vi "intersecAreaCirc.vi"(5 "theta":dbl, 6 "Recuo":dbl=130.0, 8 "error in (no error)":errorcluster, 9 "Ball/Enemy\nPosition":dbl[](array[numeric]), 10 "Game":refnum<class "Game.lvclass">, 11 "Utilities in":refnum<class "Utilities.lvclass">) -> (0 "error out":errorcluster, 2 "Position":dbl[](array[numeric]), 3 "Utilities out":refnum<class "Utilities.lvclass">)   [LabVIEW 2023, in "Utilities.lvclass"]
uses:
  Utilities.lvclass
  Game_class/Game.lvclass
  Game_class/Game.lvclass/Game.ctl
  Game_class/Read FieldRef.vi
  Field_class/Field.lvclass
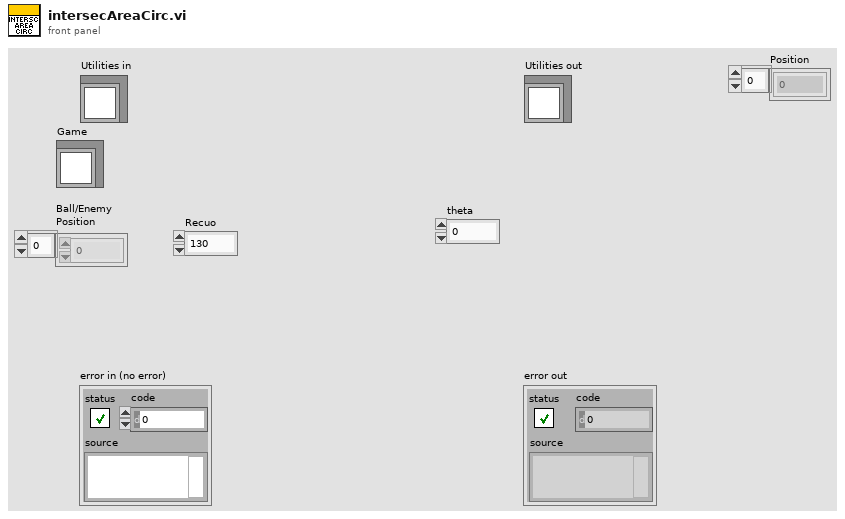
[diagram p1: front panel]
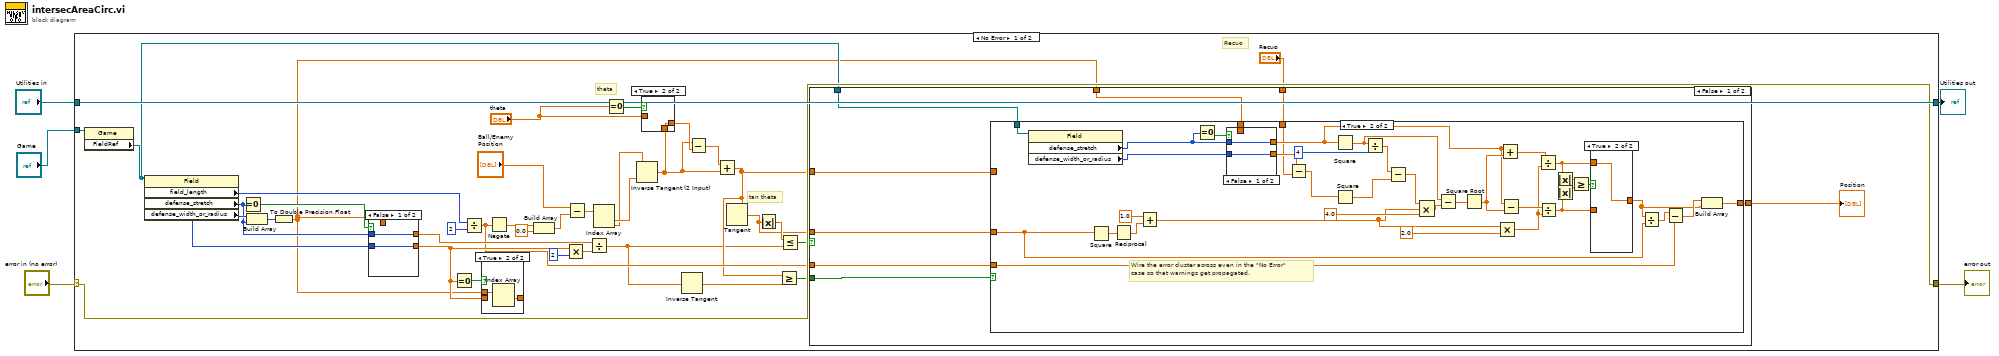
[diagram p0: block diagram]
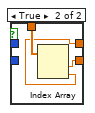
[diagram p3: hidden frame]
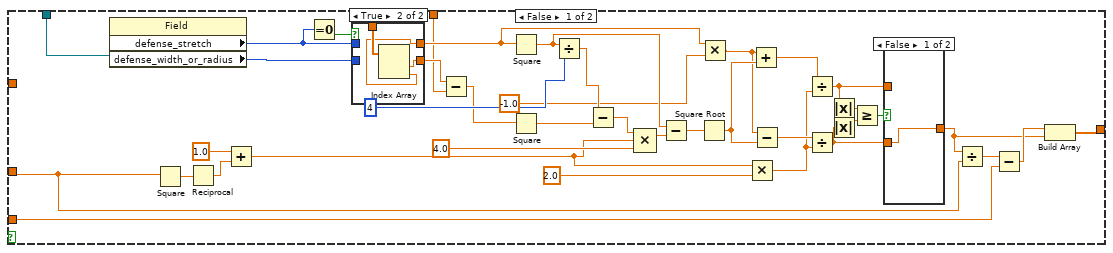
[diagram p4: hidden frame]
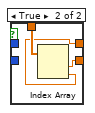
[diagram p7: hidden frame]
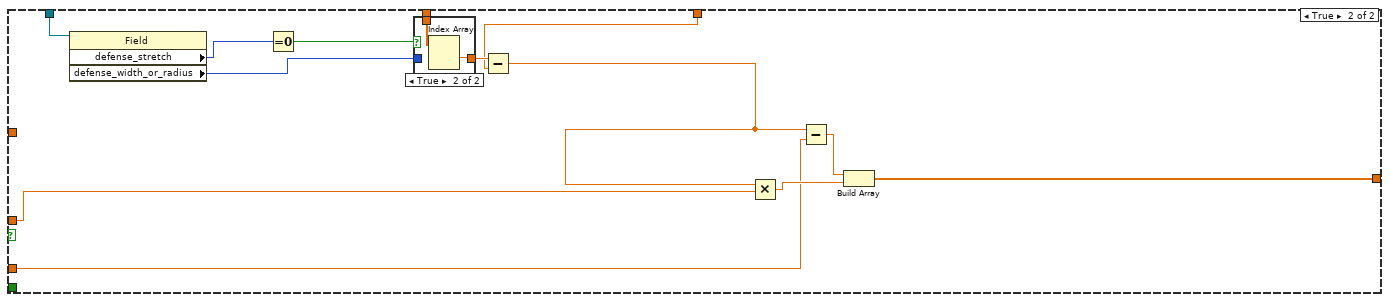
[diagram p9: hidden frame]
diagram:
  n1 = case shown="No Error" "error in (no error)" {
    selector: "error in (no error)" -> [w42 w169]
    tunnel: [w42 w169] -> w4
    tunnel: [w43 w168] -> w2
    tunnel: "Utilities in" -> [w43 w168]
    tunnel: "Game" -> [w13 _]
    frame No Error {
      # "Recuo"
      # "tan theta"
      # "theta"
      # "Wire the error cluster across even in the \"No Error\"\ncase so that warnings get propagated."
      n2 = property class="Game"(reference=w13) -> ("FieldRef"=w11:refnum<class "Field.lvclass">)  [unwired: 1 in, 2 out]
      n3 = property class="Field"(reference=w11) -> ("field_length"=w12:i32, "defense_stretch"=w9:i32, "defense_width_or_radius"=w10:i32)  [unwired: 1 in, 2 out]
      n4 = Equal To 0?(x=w9) -> (x = 0?=w38:bool)
      n5 = Build Array(w10, w9) -> (w8:i32[])
      n6 = To Double Precision Float(number=w8) -> (double precision float=w7:dbl[])
      n7 = case shown="False" w38 {
        tunnel: w9 -> [w47 _]
        tunnel: [w47 w49] -> w40
        tunnel: [w46 w48] -> w39
        tunnel: w10 -> [w46 _]
        tunnel: w7 -> [_ w50]
        frame False {
        }
        frame True {
          n8 = Index Array(array=w50) -> (element #1=w48:dbl, element #2=w49:dbl)  [unwired: 2 in]
        }
      }
      n9 = Equal To 0?(x=w39) -> (x = 0?=w25:bool)
      n10 = Divide(x=w12, y=u32 2) -> (x/y=w37:dbl)
      n11 = case shown="True" w25 {
        tunnel: [w165 w166] -> _
        tunnel: w39 -> [w165 _]
        tunnel: w7 -> [_ w167]
        frame False {
        }
        frame True {
          n12 = Index Array(array=w167) -> (element #2=w166:dbl)  [unwired: 2 in, 1 out]
        }
      }
      n13 = Negate(x=w37) -> (-x=w27:dbl)
      n14 = Build Array(w27, 0.0 ("element")) -> (w15:dbl[])
      n15 = Multiply(x=w39, y=u32 2) -> (x*y=w31:dbl)
      n16 = Subtract(x="Ball/Enemy\nPosition", y=w15) -> (x-y=w29:dbl[])
      n17 = Divide(x=w40, y=w31) -> (x/y=w17:dbl)
      n18 = Index Array(array=w29) -> (element #1=w36:dbl, element #2=w35:dbl)  [unwired: 2 in]
      n19 = Equal To 0?(x="theta") -> (x = 0?=w21:bool)
      n20 = Inverse Tangent (2 Input)(1:w36, 2:w35) -> (0:w19:dbl)
      n21 = case shown="True" w21 {
        tunnel: [w44 w45] -> w22
        tunnel: "theta" -> [w44 _]
        tunnel: w19 -> [_ w45]
        frame False {
        }
        frame True {
        }
      }
      n22 = Inverse Tangent(1:w17) -> (0:w16:dbl)
      n23 = Subtract(x=w19, y=w22) -> (x-y=w23:dbl)
      n24 = Add(x=w23, y=w19) -> (x+y=w18:dbl)
      n25 = Tangent(1:w18) -> (0:w24:dbl)
      n26 = Absolute Value(x=w24) -> (abs(x)=w30:dbl)
      n27 = Greater Or Equal?(x=w18, y=w16) -> (x >= y?=w34:bool)
      n28 = Less Or Equal?(x=w30, y=w17) -> (x <= y?=w33:bool)
      n29 = case shown="False" w33 {
        tunnel: w18 -> [w54 _]
        tunnel: [w56 w160] -> w14
        tunnel: w34 -> [w58 _]
        tunnel: w24 -> [w57 w157]
        tunnel: w37 -> [w55 w158]
        tunnel: w7 -> [w53 w153]
        tunnel: "Recuo" -> [w52 w152]
        tunnel: w11 -> [w51 w151]
        frame False {
          n30 = case shown="True" w58 {
            tunnel: w57 -> [w80 w124]
            tunnel: [w79 w123] -> w56
            tunnel: w55 -> [w75 w121]
            tunnel: w54 -> [_ _]
            tunnel: w53 -> [w70 w114]
            tunnel: w52 -> [w62 w108]
            tunnel: w51 -> [w61 w105]
            frame False {
              n31 = property class="Field"(reference=w61) -> ("defense_stretch"=w60:i32, "defense_width_or_radius"=w59:i32)  [unwired: 1 in, 2 out]
              n32 = Square(x=w80) -> (x^2=w97:dbl)
              n33 = Reciprocal(x=w97) -> (1/x=w96:dbl)
              n34 = Add(x=1.0, y=w96) -> (x+y=w83:dbl)
              n35 = Equal To 0?(x=w60) -> (x = 0?=w71:bool)
              n36 = case shown="True" w71 {
                tunnel: w60 -> [w99 _]
                tunnel: [w99 w101] -> w69
                tunnel: [w98 w100] -> w68
                tunnel: w59 -> [w98 _]
                tunnel: w70 -> [_ w102]
                frame False {
                }
                frame True {
                  n37 = Index Array(array=w102) -> (element #1=w100:dbl, element #2=w101:dbl)  [unwired: 2 in]
                }
              }
              n38 = Subtract(x=w68, y=w62) -> (x-y=w72:dbl)
              n39 = Square(x=w69) -> (x^2=w91:dbl)
              n40 = Square(x=w72) -> (x^2=w92:dbl)
              n41 = Divide(x=w91, y=u32 4) -> (x/y=w93:dbl)
              n42 = Subtract(x=w93, y=w92) -> (x-y=w89:dbl)
              n43 = Compound Arithmetic op=MULTIPLY(w89, w83, 4.0 ("value")) -> (w90:dbl)
              n44 = Subtract(x=w91, y=w90) -> (x-y=w87:dbl)
              n45 = Square Root(x=w87) -> (sqrt(x)=w86:dbl)
              n46 = Multiply(x=w69, y=-1.0) -> (x*y=w78:dbl)
              n47 = Multiply(x=w83, y=2.0) -> (x*y=w81:dbl)
              n48 = Add(x=w78, y=w86) -> (x+y=w85:dbl)
              n49 = Subtract(x=w78, y=w86) -> (x-y=w84:dbl)
              n50 = Divide(x=w85, y=w81) -> (x/y=w65:dbl)
              n51 = Divide(x=w84, y=w81) -> (x/y=w63:dbl)
              n52 = Absolute Value(x=w65) -> (abs(x)=w66:dbl)
              n53 = Absolute Value(x=w63) -> (abs(x)=w64:dbl)
              n54 = Greater Or Equal?(x=w66, y=w64) -> (x >= y?=w67:bool)
              n55 = case shown="False" w67 {
                tunnel: w63 -> [w103 _]
                tunnel: [w103 w104] -> w73
                tunnel: w65 -> [_ w104]
                frame False {
                }
                frame True {
                }
              }
              n56 = Divide(x=w73, y=w80) -> (x/y=w74:dbl)
              n57 = Subtract(x=w74, y=w75) -> (x-y=w76:dbl)
              n58 = Build Array(w76, w73) -> (w79:dbl[])
            }
            frame True {
              n59 = property class="Field"(reference=w105) -> ("defense_stretch"=w107:i32, "defense_width_or_radius"=w106:i32)  [unwired: 1 in, 2 out]
              n60 = Square(x=w124) -> (x^2=w141:dbl)
              n61 = Reciprocal(x=w141) -> (1/x=w140:dbl)
              n62 = Add(x=1.0, y=w140) -> (x+y=w127:dbl)
              n63 = Equal To 0?(x=w107) -> (x = 0?=w115:bool)
              n64 = case shown="False" w115 {
                tunnel: w107 -> [w143 _]
                tunnel: [w143 w145] -> w117
                tunnel: [w142 w144] -> w116
                tunnel: w106 -> [w142 _]
                tunnel: w114 -> [_ w146]
                frame False {
                }
                frame True {
                  n65 = Index Array(array=w146) -> (element #1=w144:dbl, element #2=w145:dbl)  [unwired: 2 in]
                }
              }
              n66 = Subtract(x=w116, y=w108) -> (x-y=w118:dbl)
              n67 = Square(x=w117) -> (x^2=w135:dbl)
              n68 = Square(x=w118) -> (x^2=w136:dbl)
              n69 = Divide(x=w135, y=u32 4) -> (x/y=w137:dbl)
              n70 = Subtract(x=w137, y=w136) -> (x-y=w133:dbl)
              n71 = Compound Arithmetic op=MULTIPLY(w133, w127, 4.0 ("value")) -> (w134:dbl)
              n72 = Subtract(x=w135, y=w134) -> (x-y=w131:dbl)
              n73 = Square Root(x=w131) -> (sqrt(x)=w130:dbl)
              n74 = Multiply(x=w127, y=2.0) -> (x*y=w125:dbl)
              n75 = Add(x=w117, y=w130) -> (x+y=w129:dbl)
              n76 = Subtract(x=w117, y=w130) -> (x-y=w128:dbl)
              n77 = Divide(x=w129, y=w125) -> (x/y=w111:dbl)
              n78 = Divide(x=w128, y=w125) -> (x/y=w110:dbl)
              n79 = Absolute Value(x=w111) -> (abs(x)=w109:dbl)
              n80 = Absolute Value(x=w110) -> (abs(x)=w113:dbl)
              n81 = Greater Or Equal?(x=w109, y=w113) -> (x >= y?=w112:bool)
              n82 = case shown="True" w112 {
                tunnel: w110 -> [w147 _]
                tunnel: [w147 w148] -> w119
                tunnel: w111 -> [_ w148]
                frame False {
                }
                frame True {
                }
              }
              n83 = Divide(x=w119, y=w124) -> (x/y=w120:dbl)
              n84 = Subtract(x=w120, y=w121) -> (x-y=w122:dbl)
              n85 = Build Array(w122, w119) -> (w123:dbl[])
            }
          }
        }
        frame True {
          n86 = property class="Field"(reference=w151) -> ("defense_stretch"=w150:i32, "defense_width_or_radius"=w149:i32)  [unwired: 1 in, 2 out]
          n87 = Equal To 0?(x=w150) -> (x = 0?=w154:bool)
          n88 = case shown="True" w154 {
            tunnel: [w162 w163] -> w155
            tunnel: w149 -> [w162 _]
            tunnel: w153 -> [_ w164]
            frame False {
            }
            frame True {
              n89 = Index Array(array=w164) -> (element #1=w163:dbl)  [unwired: 2 in, 1 out]
            }
          }
          n90 = Subtract(x=w155, y=w152) -> (x-y=w156:dbl)
          n91 = Multiply(x=w156, y=w157) -> (x*y=w161:dbl)
          n92 = Subtract(x=w156, y=w158) -> (x-y=w159:dbl)
          n93 = Build Array(w159, w161) -> (w160:dbl[])
        }
      }
      "Position" <- w14
    }
    frame Error {
    }
  }
  "error out" <- w4
  "Utilities out" <- w2
